vi "convertToKeyValuePair_integer32bit.vi"(8 "error in (no error)":errorcluster, 10 "value":i32, 11 "name":string) -> (0 "error out":errorcluster, 3 "string converted":string)   [LabVIEW 2018]
doc: "Convert an 32-bit integer numeric into a key value pair as string."
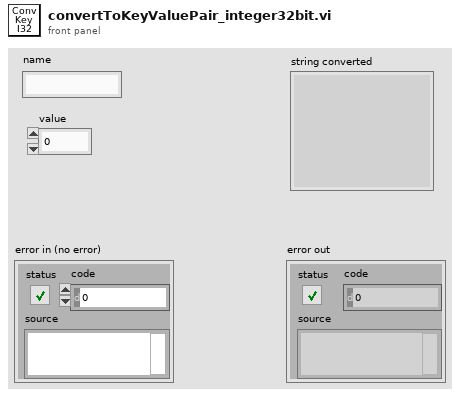
[diagram p1: front panel]
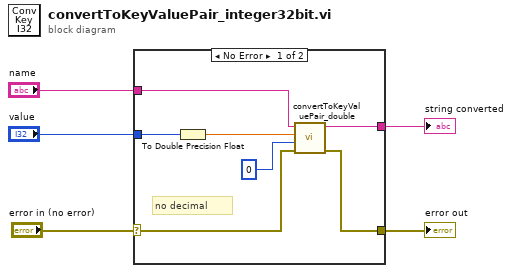
[diagram p0: block diagram]
diagram:
  n1 = case shown="No Error" "error in (no error)" {
    selector: "error in (no error)" -> [w12 w13]
    tunnel: [w10 _] -> w5
    tunnel: "value" -> [w8 _]
    tunnel: "name" -> [w7 _]
    tunnel: [w11 w13] -> w1
    frame No Error {
      # "no decimal"
      n2 = To Double Precision Float(number=w8) -> (double precision float=w6:dbl)
      n3 = call "convertToKeyValuePair_double.vi"("error in (no error)"=w12, "precision (0)"=u8 0 ("numZeros"), "value"=w6, "name"=w7) -> ("error out"=w11:errorcluster, "string converted"=w10:string)  [unwired: 6 in]
    }
    frame Error {
    }
  }
  "error out" <- w1
  "string converted" <- w5
